vi "onAddKeyValuePair.vi"(8 "error in (no error)":errorcluster, 9 "value":variant, 10 "key":string, 11 "Leaf in":refnum<class "Leaf.lvclass">) -> (0 "error out":errorcluster, 3 "Leaf out":refnum<class "Leaf.lvclass">)   [LabVIEW 2021, in "Bananas.lvlib" / "Leaf.lvclass"]
uses:
  Leaf.lvclass
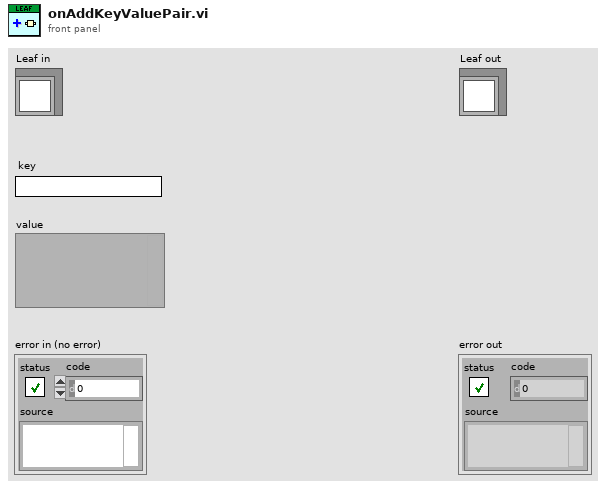
[diagram p1: front panel]
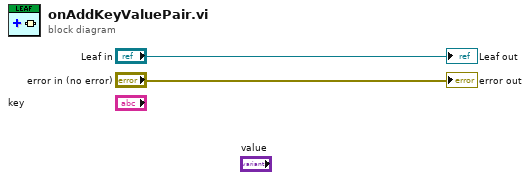
[diagram p0: block diagram]
diagram:
  "error out" <- "error in (no error)"
  "Leaf out" <- "Leaf in"
